vi "Diff Port.vi"(5 "port old":T4, 7 "port new":T4, 10 "change type":T2, 11 "refresh items in":T1[](array[typedef])) -> (3 "refresh items out":T1[](array[typedef]))   [LabVIEW 2020, in "AIM MIL-STD-1553 System Explorer.lvlib" / "Implementation.lvlib" / "Refresh.lvlib"]
uses:
  Refresh.lvlib
  Change Type.ctl
  Shared/BIU Configuration.ctl
  Shared/Address.ctl
  Shared/Major Frame Definition.ctl
  Shared/Minor Frame Definition.ctl
  Shared/Message Definition.ctl
  Shared/Message Type.ctl
  Shared/Terminal Endpoint.ctl
  Shared/Parameter Definition.ctl
  MCL Row.ctl
  Symbols.ctl
  Name to Symbol.vi
  Scripting/Constants.vi
  Scripting/AIM MIL-STD-1553 Scripting.lvlib
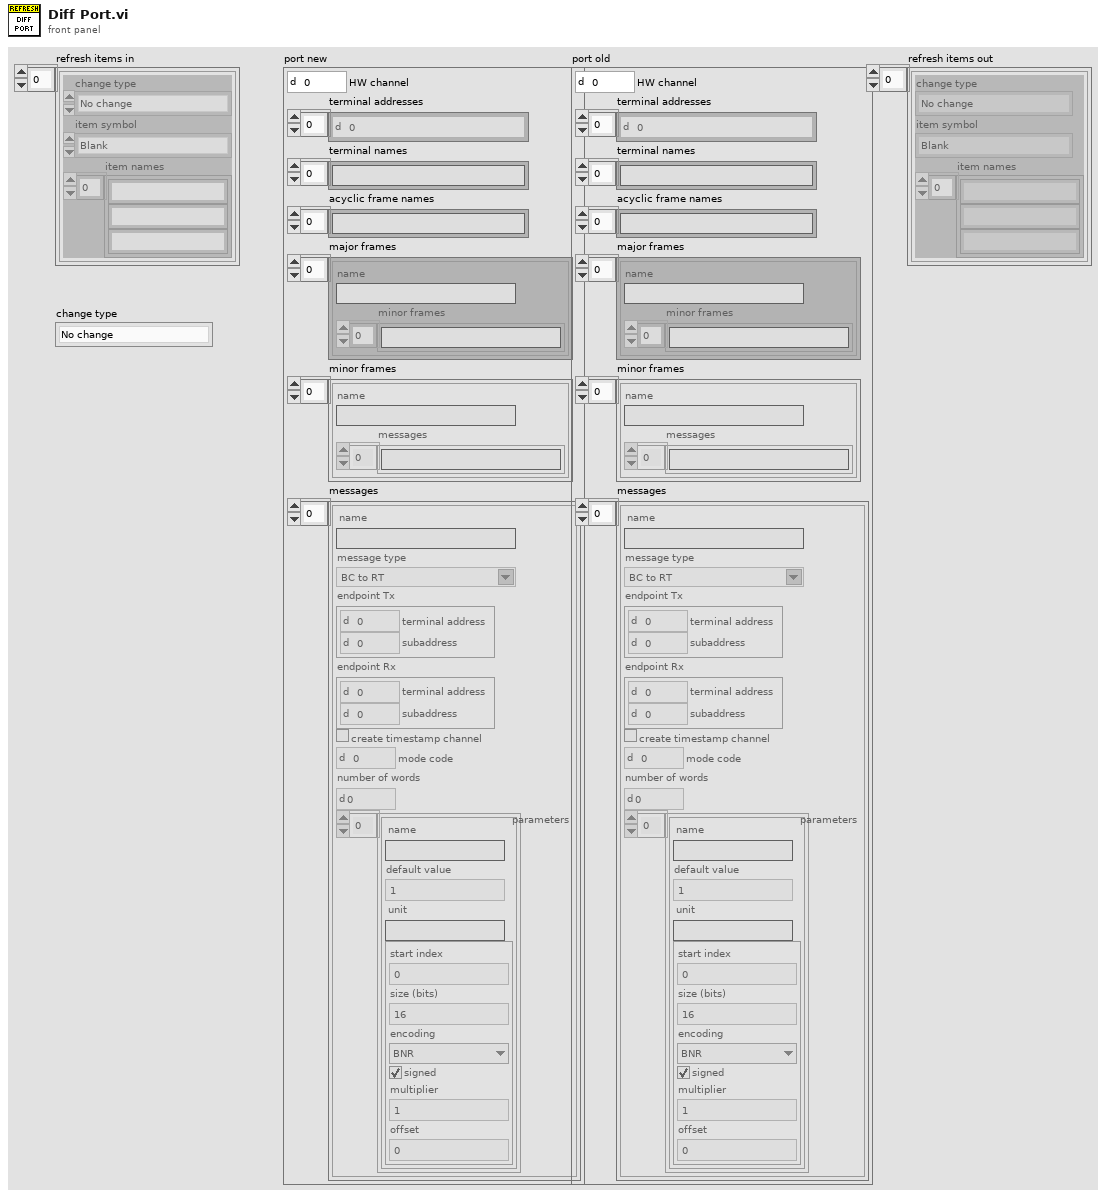
[diagram p1: front panel]
types:
  T1 = typedef "AIM MIL-STD-1553 System Explorer.lvlib/Implementation.lvlib/Refresh.lvlib/MCL Row.ctl" = cluster{"change type":T2, "item symbol":T3, "item names":string[]}
  T2 = typedef "AIM MIL-STD-1553 System Explorer.lvlib/Implementation.lvlib/Refresh.lvlib/Change Type.ctl" = enum16{"No change", "Modify", "Add", "Remove"}
  T3 = typedef "AIM MIL-STD-1553 System Explorer.lvlib/Implementation.lvlib/Refresh.lvlib/Symbols.ctl" = enum16{"Blank", "MIL-STD-1553", "Port", "Remote Terminal", "Subaddress", "Bus Controller", "Acyclic Frame", "Mode Code", "Message", "Parameter", "Item"}
  T4 = typedef "BIU Configuration.ctl" = cluster{"HW channel":u16, "terminal addresses":T5[], "terminal names":string[], "acyclic frame names":string[], "major frames":T6[], "minor frames":T7[], "messages":T8[]}
  T5 = typedef "Address.ctl" = u16
  T6 = typedef "Major Frame Definition.ctl" = cluster{"name":string, "minor frames":string[]}
  T7 = typedef "Minor Frame Definition.ctl" = cluster{"name":string, "messages":string[]}
  T8 = typedef "Message Definition.ctl" = cluster{"name":string, "message type":T9, "endpoint Tx":T10, "endpoint Rx":T10, "create timestamp channel":bool, "mode code":u16, "number of words":u16, "parameters":cluster{"name":string, "default value":dbl, "unit":string, "parameter definition":T11}[]}
  T9 = typedef "Message Type.ctl" = string
  T10 = typedef "Terminal Endpoint.ctl" = cluster{"terminal address":T5, "subaddress":T5}
  T11 = typedef "Parameter Definition.ctl" = cluster{"start index":i32, "size (bits)":i32, "encoding":enum16{"BNR", "BCD", "Discrete"}, "signed":bool, "multiplier":dbl, "offset":dbl}
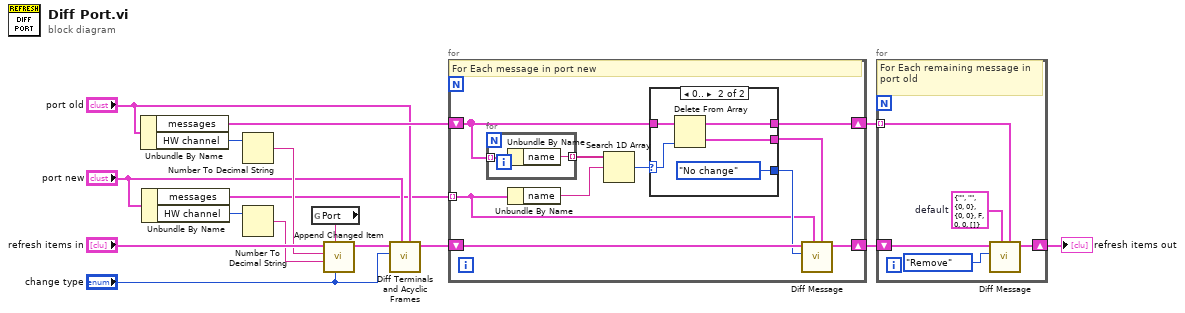
[diagram p0: block diagram]
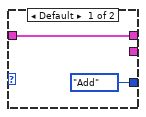
[diagram p2: hidden frame]
diagram:
  n1 = Unbundle By Name("port old") -> ("messages"=w7:T8[], "HW channel"=w14:u16)
  n2 = Unbundle By Name("port new") -> ("messages"=w1:T8[], "HW channel"=w13:u16)
  n3 = Number To Decimal String(number=w14) -> (decimal integer string=w12:string)  [unwired: 1 in]
  n4 = Number To Decimal String(number=w13) -> (decimal integer string=w11:string)  [unwired: 1 in]
  n5 = global read "Constants.vi" "Port"() -> (w16:string)
  n6 = call "Append Changed Item.vi"("change type"="change type", "item name"=w16, "new value"=w11, "old value"=w12, "refresh items in"="refresh items in") -> ("refresh items out"=w10:T1[])  [unwired: 5 in, 1 out]
  n7 = call "Diff Terminals and Acyclic Frames.vi"("port old"="port old", "port new"="port new", "change type"="change type", "refresh items in"=w10) -> ("refresh items out"=w8:T1[])  [unwired: 7 in]
  n8 = for {
    tunnel: w1 -> [w17] mode=indexing
    shift-right: [w23] -> w5
    shift-left: w7 -> [w24]
    shift-right: [w21] -> w4
    shift-left: w8 -> [w20]
    # "For Each message in port new"
    n9 = for {
      tunnel: w24 -> [w35] mode=indexing
      tunnel: [w34] -> w25 mode=indexing
      n10 = Unbundle By Name(w35) -> ("name"=w34:string)
    }
    n11 = Unbundle By Name(w17) -> ("name"=w22:string)
    n12 = Search 1D Array(1D array=w25, element=w22) -> (index of element=w26:i32)  [unwired: 1 in]
    n13 = case shown="0.." w26 {
      selector: w26 -> [_ w31]
      tunnel: w24 -> [w28 w33]
      tunnel: [w28 w32] -> w23
      tunnel: [_ w30] -> w19
      tunnel: [Change_Type."Add" ("change type") Change_Type."No change" ("change type")] -> w18
      frame Default {
      }
      frame 0.. {
        n14 = Delete From Array(array=w33, index=w31) -> (deleted portion=w30:T8, array with subset deleted=w32:T8[])  [unwired: 1 in]
      }
    }
    n15 = call "Diff Message.vi"("message old"=w19, "message new"=w17, "change type"=w18, "refresh items in"=w20) -> ("refresh items out"=w21:T1[])  [unwired: 7 in]
  }
  n16 = for {
    shift-right: [w40] -> w6
    shift-left: w4 -> [w39]
    tunnel: w5 -> [w37] mode=indexing
    w36 = T8 {"name"="", "message type"="", "endpoint Tx"={"terminal address"=0, "subaddress"=0}, "endpoint Rx"={"terminal address"=0, "subaddress"=0}, "create timestamp channel"=FALSE, "mode code"=0, "number of words"=0, "parameters"=[]}  # default
    # "For Each remaining message in port old"
    n17 = call "Diff Message.vi"("message old"=w37, "message new"=w36, "change type"=Change_Type."Remove", "refresh items in"=w39) -> ("refresh items out"=w40:T1[])  [unwired: 7 in]
  }
  "refresh items out" <- w6
